vi "Count Color.vi"() -> (0 "Completed":bool)   [LabVIEW 2019]
uses:
  Robot Global Data.vi
panel:
  in  "Nb Changements pour valider":dbl=26.0
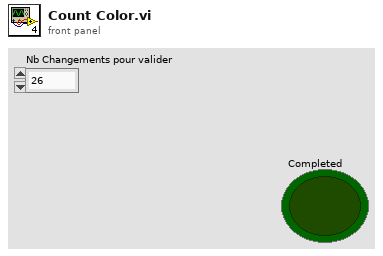
[diagram p1: front panel]
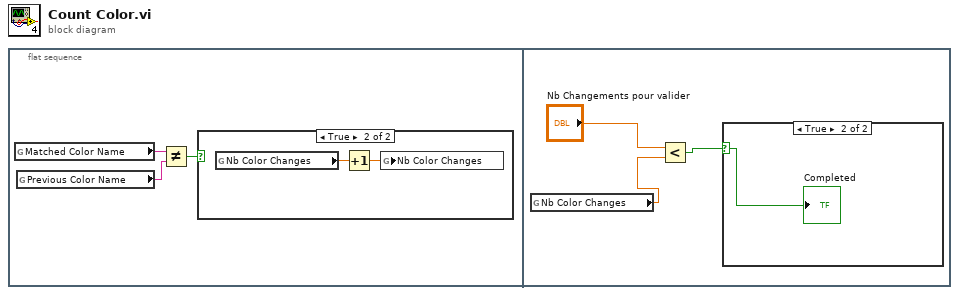
[diagram p0: block diagram]
diagram:
  n1 = flat-sequence {
    frame #0 {
      n2 = global read "Robot Global Data.vi" "Matched Color Name"() -> (w2:string)
      n3 = global read "Robot Global Data.vi" "Previous Color Name"() -> (w3:string)
      n4 = Not Equal?(x=w2, y=w3) -> (x != y?=w1:bool)
      n5 = case shown="True" w1 {
        frame False {
        }
        frame True {
          n6 = global read "Robot Global Data.vi" "Nb Color Changes"() -> (w4:dbl)
          n7 = Increment(x=w4) -> (x+1=w5:dbl)
          n8 = global write "Robot Global Data.vi" "Nb Color Changes"(w5) -> ()
        }
      }
    }
    frame #1 {
      n9 = global read "Robot Global Data.vi" "Nb Color Changes"() -> (w7:dbl)
      n10 = Less?(x="Nb Changements pour valider", y=w7) -> (x < y?=w6:bool)
      n11 = case shown="True" w6 {
        selector: w6 -> [_ w9]
        frame False {
        }
        frame True {
          "Completed" <- w9
        }
      }
    }
  }
